vi "ReadVacuumSwitches - Copy.vi"(3 "error in":errorcluster) -> (5 "OutVacStatus":u32, 6 "data":bool[](array[boolean]) caption="VacuumStatusBool", 7 "error out":errorcluster)   [LabVIEW 2019]
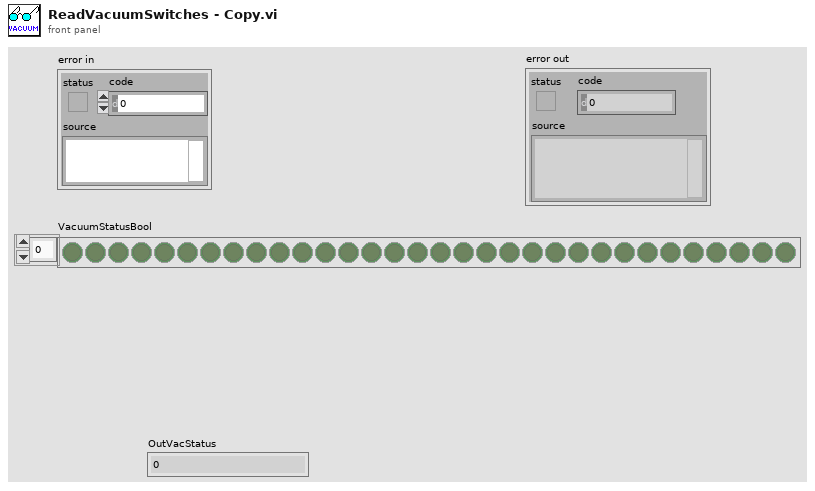
[diagram p1: front panel]
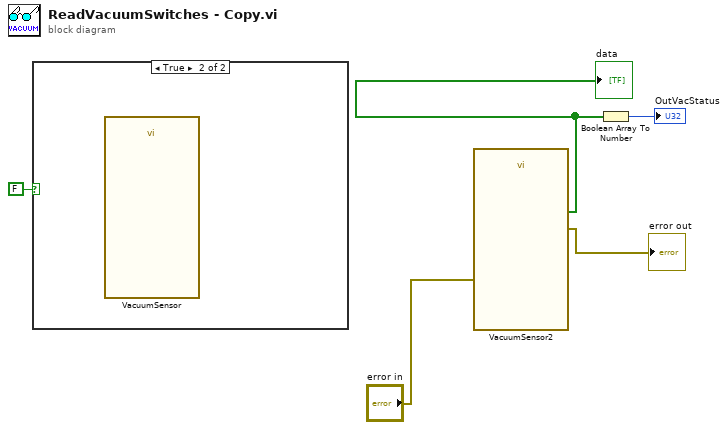
[diagram p0: block diagram]
diagram:
  n1 = case shown="True" FALSE {
    frame False {
    }
    frame True {
      n2 = call "VacuumSensor"() -> ()  [unwired: 17 in, 3 out]
    }
  }
  n3 = call "VacuumSensor2"("error in"="error in") -> ("data"=w1:bool[], "error out"=→"error out":errorcluster)  [unwired: 16 in, 1 out]
  "data" <- w1
  n4 = Boolean Array To Number(Boolean array=w1) -> (number=→"OutVacStatus":u32)
